vi "APC_9049_KnockCA50Control.vi"(0 "Knock control?":bool, 3 "CA50 control?":bool=TRUE, 4 "Manual SA [CADBTDC]":dbl=-60.0, 5 "CA50setpoint [CADATDC]":dbl format="%.2f") -> (1 "SA [CADBTDC]":dbl format="%.2f")   [LabVIEW 2020]
uses:
  <vilib>/addons/control/pid/pid.llb/PID Advanced (DBL).vi
  <vilib>/addons/control/pid/NI_PID_pid.lvlib
panel:
  in  "Advance (no knock)":dbl
  in  "Delay by knock":dbl
  out "Sensed knock":bool
  in  "SA range [CADBTDC]":cluster{"output high":dbl, "output low":dbl}={"output high"=100.0, "output low"=-100.0} {"output low" format="%.2f"; "output high" format="%.2f"}
  in  "reinitialize? (F)":bool
  in  "PID gains":T1={"proportional gain (Kc)"=1.0, "integral time (Ti, min)"=0.01, "derivative time (Td, min)"=0.0} {"derivative time (Td, min)" format="%.3f"; "integral time (Ti, min)" format="%.3f"; "proportional gain (Kc)" format="%.3f"}
  in  "CA50 range [CADBTDC]":cluster{"setpoint high":dbl, "setpoint low":dbl}={"setpoint high"=100.0, "setpoint low"=0.0} {"setpoint high" format="%.2f"; "setpoint low" format="%.2f"}
  out "CA50 key cylinder [CADATDC]":dbl format="%.2f"
  # "NOTE: CADBTDC"
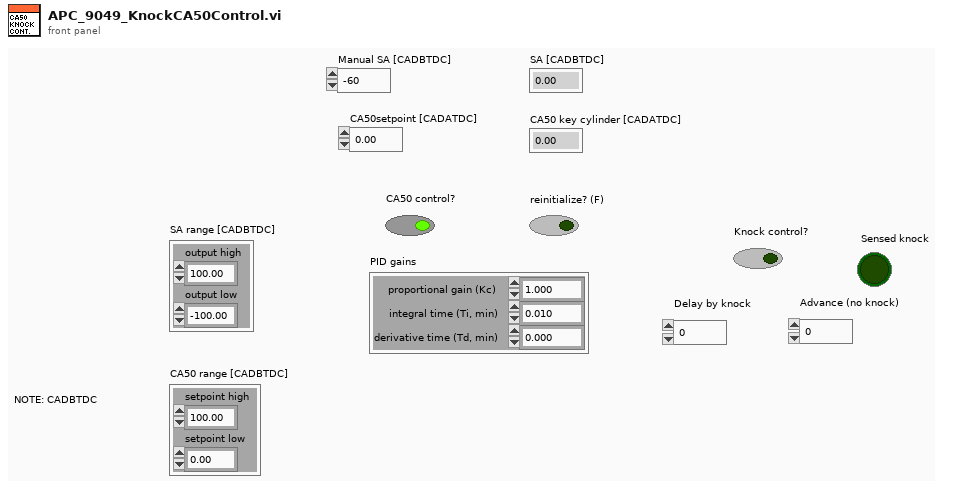
[diagram p1: front panel]
types:
  T1 = cluster{"proportional gain (Kc)":dbl, "integral time (Ti, min)":dbl, "derivative time (Td, min)":dbl}
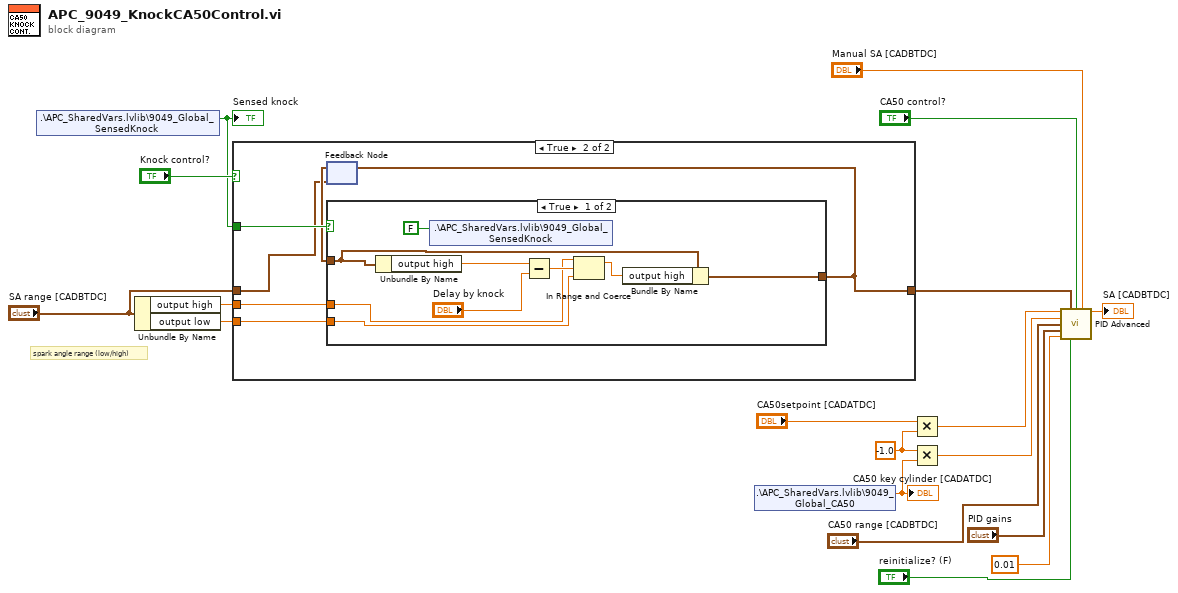
[diagram p0: block diagram]
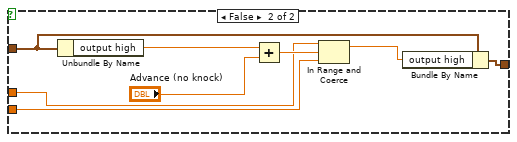
[diagram p3: hidden frame]
diagram:
  w2 = -1.0 ("x")
  # "spark angle range (low/high)"
  n1 = shared-variable ".\\APC_SharedVars.lvlib\\9049_Global_SensedKnock"() -> (w3:bool)  [unwired: 1 in, 1 out]
  "Sensed knock" <- w3
  n2 = Unbundle By Name("SA range [CADBTDC]") -> ("output high"=w5:dbl, "output low"=w4:dbl)
  n3 = case shown="True" "Knock control?" {
    tunnel: w3 -> [_ w25]
    tunnel: "SA range [CADBTDC]" -> [w19 w23]
    tunnel: [w19 w22] -> w11
    tunnel: w5 -> [_ w21]
    tunnel: w4 -> [_ w20]
    frame False {
    }
    frame True {
      n4 = feedback #1(w23) -> (w24:cluster{"output high":dbl, "output low":dbl})
      n5 = case shown="True" w25 {
        tunnel: w24 -> [w34 w42]
        tunnel: [w33 w41] -> w22
        tunnel: w21 -> [w28 w36]
        tunnel: w20 -> [w27 w35]
        frame True {
          n6 = Unbundle By Name(w34) -> ("output high"=w32:dbl)
          n7 = shared-variable ".\\APC_SharedVars.lvlib\\9049_Global_SensedKnock"(FALSE ("Sensed knock")) -> ()  [unwired: 1 in, 1 out]
          n8 = Subtract(x=w32, y="Delay by knock") -> (x-y=w29:dbl)
          n9 = In Range and Coerce(upper limit=w28, x=w29, lower limit=w27) -> (coerced(x)=w30:dbl)  [unwired: 1 out]
          n10 = Bundle By Name(cluster=w34, "output high"=w30) -> (w33:cluster{"output high":dbl, "output low":dbl})
        }
        frame False {
          n11 = Unbundle By Name(w42) -> ("output high"=w40:dbl)
          n12 = Add(x=w40, y="Advance (no knock)") -> (x+y=w38:dbl)
          n13 = In Range and Coerce(upper limit=w36, x=w38, lower limit=w35) -> (coerced(x)=w37:dbl)  [unwired: 1 out]
          n14 = Bundle By Name(cluster=w42, "output high"=w37) -> (w41:cluster{"output high":dbl, "output low":dbl})
        }
      }
      n15 = feedback-in #1(w22) -> ()
    }
  }
  n16 = shared-variable ".\\APC_SharedVars.lvlib\\9049_Global_CA50"() -> (w1:dbl)  [unwired: 1 in, 1 out]
  "CA50 key cylinder [CADATDC]" <- w1
  n17 = Multiply(x="CA50setpoint [CADATDC]", y=w2) -> (x*y=w8:dbl)
  n18 = Multiply(x=w2, y=w1) -> (x*y=w7:dbl)
  n19 = call-poly <vilib>:"PID Advanced.vi"("setpoint"=w8, "output range"=w11, "auto? (T)"="CA50 control?", "manual control"="Manual SA [CADBTDC]", "process variable"=w7, "setpoint range"="CA50 range [CADBTDC]", "PID gains"="PID gains", "dt (s)"=0.01, "reinitialize? (F)"="reinitialize? (F)") -> ("output"=→"SA [CADBTDC]":dbl)  [unwired: 5 in, 1 out]
